vi "GetTerms3.vi"(0 "XRef":T10, 1 "State In":T9) -> (14 "Terms":T1)   [LabVIEW 2018, in "OpenG Reverse 2D Array.xnode"]
doc: "This ability VI is used to describe your terminals to LabVIEW. Terms is an array of clusters describing the XNode's terminals.\n ID: A unique string identifying the terminal.\n Name: The name of the terminal visible to the user. Remember to localize it.\n Type: The data type of the terminal (as a Variant). The data put in the variant will be used as the default for the input terminal if it's left unwired.\n Bounds: A rectangle defining the bounds of the terminal relative to the bounds of the XNode. The bounds must be within the bounds of the XNode, and for whiskers to draw properly, they must be flush with at least one side of the XNode.\n Input?: Indicates whether or not this terminals is an input.\n Required?: Indicates whether the user must wire this terminal for the XNode to not be broken. Ignored on outputs.\n Recommended?: Indicates whether the terminal is recommended.\n Hidden?: Indicates whether the terminal is hidden. When a terminal is hidden, it cannot be wired to via user interaction or scripting. However, if it is already wired to when the hidden flag is changed to true, it will remain wired.\n Adaptive?: Indicates that the term should change to match the type of its source if it is wired.\n Direction?: Indicates what direction the wire stub should point. Choose auto to let LV decide based on the terms bounds being on the nodes edge.\n \n The IDs are used by LabVIEW to keep track of your terminals. When you respecify your terminals, LabVIEW can tell whther terminals are new, deleted, or moved by the unique IDs. The order is irrelevant. If you move a terminal, then any wire connected to it will move with it.\n \n If you want to update your terminals, you should return the UpdateTerms reply in one of your ability VIs.\n\nDefault behavior: None.\n\nThis ability does not provide UI and OS messages are not handled."
uses:
  OpenG Reverse 2D Array.xnode
  <vilib>/XNodeSupport/XNodeXNodeRef.ctl
  State.ctl
  <vilib>/XNodeSupport/XNodeTerm3Array.ctl
  <vilib>/XNodeSupport/XNodeTerm3.ctl
  <vilib>/XNodeSupport/XNodeString.ctl
  <vilib>/XNodeSupport/XNodeVariant.ctl
  <vilib>/XNodeSupport/XNodeRect32.ctl
  <vilib>/XNodeSupport/XNodeInt.ctl
  <vilib>/XNodeSupport/XNodeBool.ctl
  <vilib>/XNodeSupport/XNodeTermDirection.ctl
  <vilib>/XNodeSupport/NI_XNodeSupport.lvlib
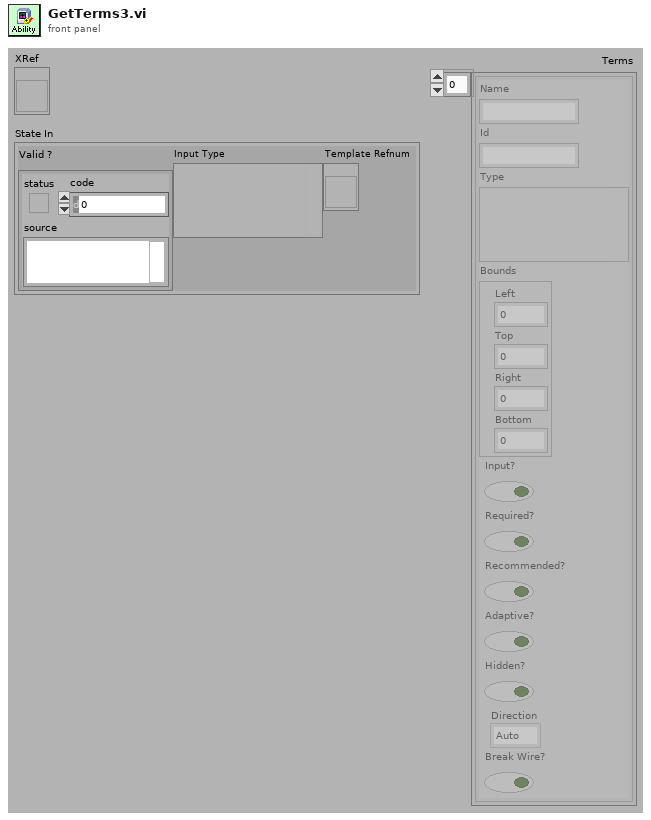
[diagram p1: front panel]
types:
  T1 = typedef "NI_XNodeSupport.lvlib/XNodeTerm3Array.ctl" = T2[]
  T2 = typedef "NI_XNodeSupport.lvlib/XNodeTerm3.ctl" = cluster{"Name":T3, "Id":T3, "Type":T4, "Bounds":T5, "Input?":T7, "Required?":T7, "Recommended?":T7, "Adaptive?":T7, "Hidden?":T7, "Direction":T8, "Break Wire?":T7}
  T3 = typedef "NI_XNodeSupport.lvlib/XNodeString.ctl" = string
  T4 = typedef "NI_XNodeSupport.lvlib/XNodeVariant.ctl" = variant
  T5 = typedef "NI_XNodeSupport.lvlib/XNodeRect32.ctl" = cluster{"Left":T6, "Top":T6, "Right":T6, "Bottom":T6}
  T6 = typedef "NI_XNodeSupport.lvlib/XNodeInt.ctl" = i32
  T7 = typedef "NI_XNodeSupport.lvlib/XNodeBool.ctl" = bool
  T8 = typedef "NI_XNodeSupport.lvlib/XNodeTermDirection.ctl" = enum32{"Auto", "Up", "Down", "Left", "Right", "Center"}
  T9 = typedef "OpenG Reverse 2D Array.xnode/State.ctl" = cluster{"Valid ?":errorcluster, "Input Type":variant, "Template Refnum":refnum<vi>}
  T10 = typedef "NI_XNodeSupport.lvlib/XNodeXNodeRef.ctl" = refnum<vi>
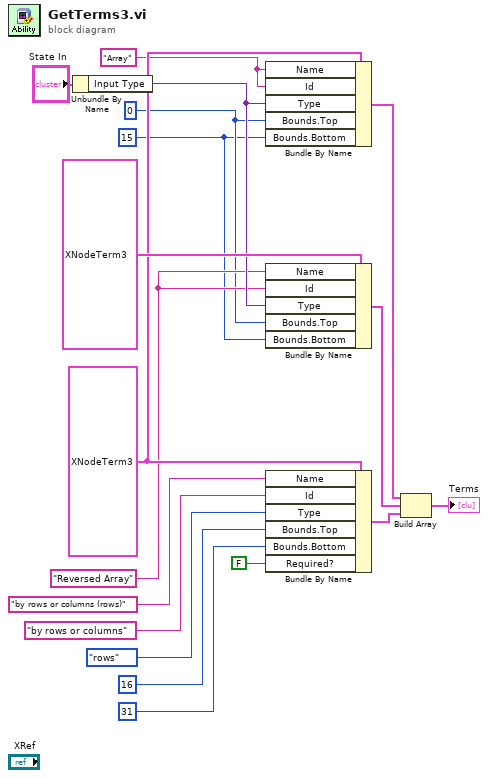
[diagram p0: block diagram]
diagram:
  w8 = T6 15 ("Bounds.Bottom")
  w9 = T6 0 ("Bounds.Top")
  w10 = T3 "Reversed Array" ("Name")
  w13 = T3 "Array" ("Name")
  w14 = T2 {"Name"="Inputs", "Id"="", "Type"=variant, "Bounds"={"Left"=0, "Top"=0, "Right"=15, "Bottom"=0}, "Input?"=TRUE, "Required?"=TRUE, "Recommended?"=TRUE, "Adaptive?"=FALSE, "Hidden?"=FALSE, "Direction"=enum."Left", "Break Wire?"=FALSE} ("Term 3")
  n1 = Unbundle By Name("State In") -> ("Input Type"=w11:variant)
  n2 = Bundle By Name(cluster=w14, "Name"=w13, "Id"=w13, "Type"=w11, "Bounds.Top"=w9, "Bounds.Bottom"=w8) -> (w17:T2)
  n3 = Bundle By Name(cluster=T2 {"Name"="Outputs", "Id"="", "Type"=variant, "Bounds"={"Left"=16, "Top"=0, "Right"=32, "Bottom"=0}, "Input?"=FALSE, "Required?"=FALSE, "Recommended?"=TRUE, "Adaptive?"=FALSE, "Hidden?"=FALSE, "Direction"=enum."Right", "Break Wire?"=FALSE} ("Term 3"), "Name"=w10, "Id"=w10, "Type"=w11, "Bounds.Top"=w9, "Bounds.Bottom"=w8) -> (w16:T2)
  n4 = Bundle By Name(cluster=w14, "Name"=T3 "by rows or columns (rows)", "Id"=T3 "by rows or columns", "Type"=enum16{"rows", "columns"}."rows" ("by rows or columns (rows)"), "Bounds.Top"=T6 16, "Bounds.Bottom"=T6 31, "Required?"=T7 FALSE) -> (w2:T2)
  n5 = Build Array(w17, w16, w2) -> (→"Terms":T2[])
